vi "Class VI Children Data.vi"(7 "Destination":path, 8 "Error In":errorcluster, 11 "Class In":refnum<vi>) -> (0 "Error Out":errorcluster, 2 "Data":refnum<class "Map.lvclass">[](array[class]), 3 "Class Out":refnum<vi>)   [LabVIEW 2018, in "Scripts.lvlib"]
uses:
  Scripts.lvlib
  Toolkit/Data/Map/Map.lvclass
  Toolkit/Data/Pair/Support/From String.vi
  Toolkit/Data/Map/Support/From Pair Array.vi
  Toolkit/Data/Pair/Pair.lvclass
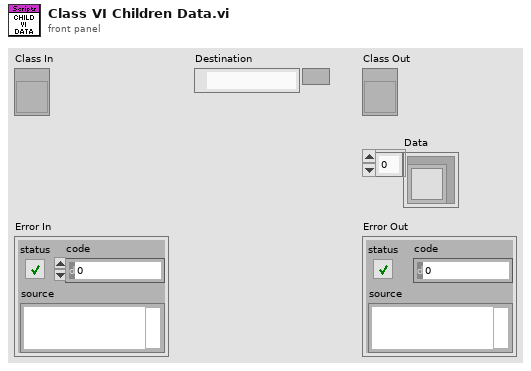
[diagram p1: front panel]
types:
  T1 = enum32{"invalid scope", "public", "private", "protected", "community"}
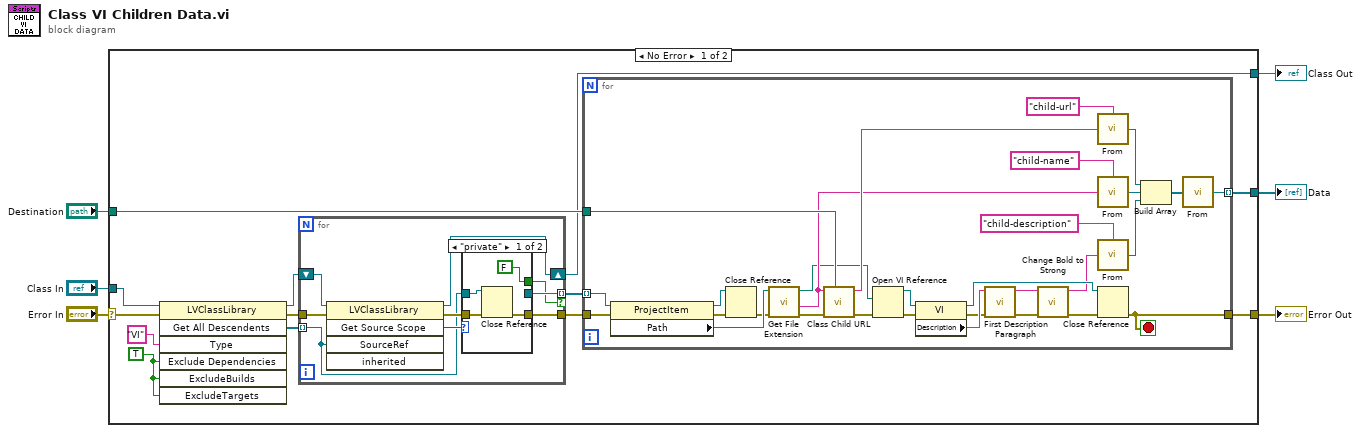
[diagram p0: block diagram]
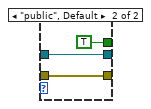
[diagram p2: hidden frame]
diagram:
  n1 = case shown="No Error" "Error In" {
    selector: "Error In" -> [w15 w67]
    tunnel: [w19 w67] -> w6
    tunnel: "Destination" -> [w17 _]
    tunnel: "Class In" -> [w16 w66]
    tunnel: [w11 w66] -> w1
    tunnel: [w18 _] -> w4
    frame No Error {
      w13 = TRUE ("ExcludeDependencies")
      n2 = invoke class="LVClassLibrary" method="Get All Descendents"(reference=w16, error in=w15, "Type"="VI", "Exclude Dependencies"=w13, "ExcludeBuilds"=w13, "ExcludeTargets"=w13) -> (reference out=w12:refnum<vi>, error out=w10:errorcluster, "All Descendents"=w8:refnum<vi>[])  [unwired: 1 in, 4 out]
      n3 = for {
        shift-right: [w27] -> w11
        shift-left: w12 -> [w28]
        tunnel: w10 -> [w26]
        tunnel: [w20] -> w9
        tunnel: w8 -> [w23] mode=indexing
        tunnel: [w22] -> w7 mode=indexing if=w21
        n4 = invoke class="LVClassLibrary" method="Get Source Scope"(reference=w28, error in=w26, "SourceRef"=w23) -> (reference out=w27:refnum<vi>, error out=w24:errorcluster, "GetSourceScope"=w25:T1)  [unwired: 2 in, 2 out]
        n5 = case shown="\"private\"" w25 {
          tunnel: w24 -> [w32 w35]
          tunnel: w23 -> [w31 w34]
          tunnel: [w29 w35] -> w20
          tunnel: [_ w34] -> w22
          tunnel: [FALSE TRUE] -> w21
          frame "private" {
            n6 = Close Reference(reference=w31, error in (no error)=w32) -> (error out=w29:errorcluster)
          }
          frame "public", Default {
          }
        }
      }
      n7 = for {
        tunnel: w9 -> [w59]
        tunnel: [w60] -> w18 mode=indexing
        tunnel: [w51] -> w19
        tunnel: w17 -> [w47]
        tunnel: w7 -> [w42] mode=indexing
        stop <- w51 stop-if-true
        n8 = property class="ProjectItem"(reference=w42, error in=w59) -> (reference out=w55:refnum<vi>, error out=w56:errorcluster, "Path"=w54:path)
        n9 = Close Reference(reference=w55, error in (no error)=w56) -> (error out=w53:errorcluster)
        n10 = call <vilib>:"Get File Extension.vi"("error in (no error)"=w53, "file"=w54) -> ("error out"=w50:errorcluster, "filename without extension"=w46:string, "dup file"=w40:path)  [unwired: 5 in, 2 out]
        n11 = call "Class Child URL.vi"("Destination"=w47, "Error In"=w50, "Name"=w46) -> ("Error Out"=w49:errorcluster, "Child URL"=w48:string)  [unwired: 7 in]
        n12 = Open VI Reference(vi path=w40, error in (no error)=w49) -> (vi reference=w39:refnum<vi>, error out=w41:errorcluster)  [unwired: 4 in]
        n13 = property class="VI"(reference=w39, error in=w41) -> (reference out=w52:refnum<vi>, error out=w37:errorcluster, "Description"=w45:string)
        n14 = call "First Description Paragraph.vi"("Error In"=w37, "Description"=w45) -> ("Error Out"=w36:errorcluster, "First Paragraph"=w38:string)  [unwired: 8 in]
        n15 = call "Change Bold to Strong.vi"("Error In"=w36, "Bold Description"=w38) -> ("Error Out"=w44:errorcluster, "Strong Description"=w43:string)  [unwired: 8 in]
        n16 = call-poly "From.vi"("Value"=w48, "Key"="child-url") -> ("Pair"=w63:refnum<class "Pair.lvclass">)
        n17 = call-poly "From.vi"("Value"=w46, "Key"="child-name") -> ("Pair"=w62:refnum<class "Pair.lvclass">)
        n18 = call-poly "From.vi"("Value"=w43, "Key"="child-description") -> ("Pair"=w57:refnum<class "Pair.lvclass">)
        n19 = Close Reference(reference=w52, error in (no error)=w44) -> (error out=w51:errorcluster)
        n20 = Build Array(w63, w62, w57) -> (w61:refnum<class "Pair.lvclass">[])
        n21 = call-poly "From.vi"("Pairs"=w61) -> ("Map"=w60:refnum<class "Map.lvclass">)  [unwired: 1 in]
      }
    }
    frame Error {
    }
  }
  "Error Out" <- w6
  "Data" <- w4
  "Class Out" <- w1
